vi "Barcode 001 Time.vi"(8 "error in (no error)":errorcluster, 11 "Code":string) -> (0 "error out":errorcluster, 3 "Code out":string)   [LabVIEW 2014]
panel:
  in  "s":bool
  in  "day of month":i32
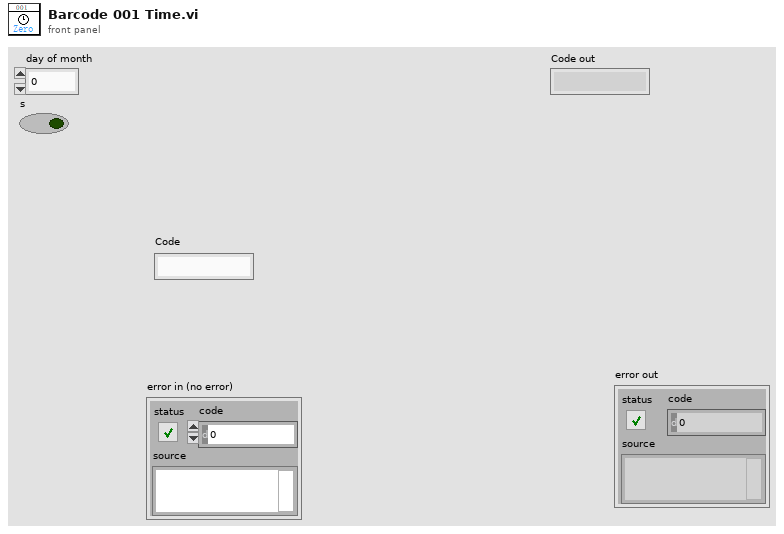
[diagram p1: front panel]
types:
  T1 = typedef "LVDateTimeRec.ctl" = cluster{"fractional second":dbl, "second":i32, "minute":i32, "hour":i32, "day of month":i32, "month":i32, "year":i32, "day of week":i32, "day of year":i32, "DST":i32}
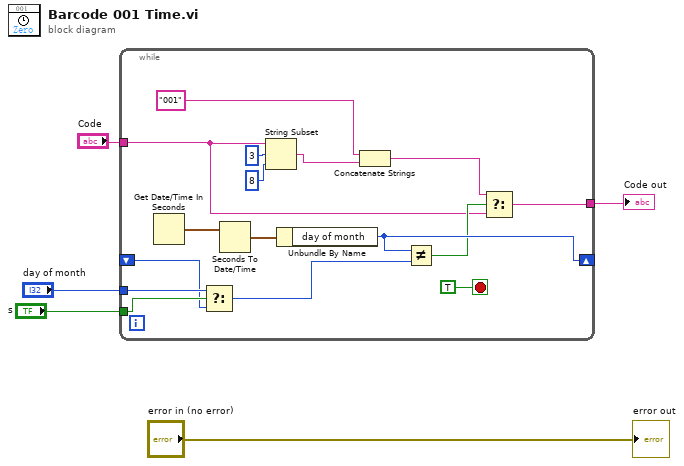
[diagram p0: block diagram]
diagram:
  n1 = while {
    shift-right: [w13] -> _
    shift-left: _ -> [w7]
    tunnel: "Code" -> [w11]
    tunnel: [w10] -> w3
    tunnel: "day of month" -> [w9]
    tunnel: "s" -> [w8]
    stop <- TRUE stop-if-true
    n2 = Get Date/Time In Seconds() -> (seconds since 1Jan1904=w14:timestamp)
    n3 = Select(t=w9, s=w8, f=w7) -> (s? t:f=w6:i32)
    n4 = Seconds To Date/Time(time stamp (now)=w14) -> (date time rec=w15:T1)  [unwired: 1 in]
    n5 = String Subset(string=w11, offset (0)=3, length (rest)=8 ("length (rest)")) -> (substring=w19:string)
    n6 = Unbundle By Name(w15) -> ("day of month"=w13:i32)
    n7 = Concatenate Strings("001", w19) -> (w18:string)
    n8 = Not Equal?(x=w13, y=w6) -> (x != y?=w12:bool)
    n9 = Select(t=w18, s=w12, f=w11) -> (s? t:f=w10:string)
  }
  "Code out" <- w3
  "error out" <- "error in (no error)"
